vi "NI9205_SUB-VI_STALLDATA.vi"(7 "milliseconds to wait":u32=100, 8 "error in (no error)":errorcluster) -> (0 "error out":errorcluster)   [LabVIEW 2020]
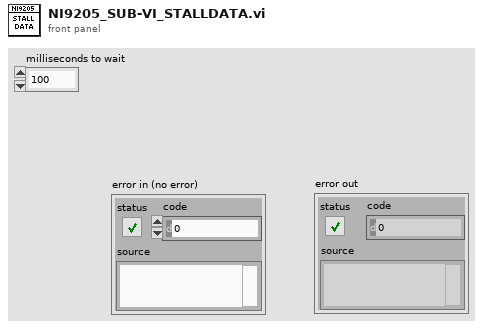
[diagram p1: front panel]
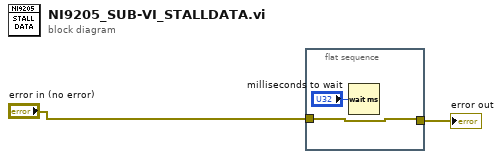
[diagram p0: block diagram]
diagram:
  n1 = flat-sequence {
    tunnel: "error in (no error)" -> [w3]
    tunnel: [w3] -> w1
    frame #0 {
      n2 = Wait (ms)(milliseconds to wait="milliseconds to wait") -> ()  [unwired: 1 out]
    }
  }
  "error out" <- w1
